vi "GetText.vi"(8 "error in":errorcluster, 11 "node in":refnum<class "Run VI Node.lvclass">) -> (0 "error out":errorcluster, 1 "additional text":string, 2 "text":string, 3 "node out":refnum<class "Run VI Node.lvclass">, 4 "glyph":string)   [LabVIEW 2014, in "Run VI Node.lvclass"]
doc: "Returns the text representation of the node used for the tree control."
uses:
  Run VI Node.lvclass
  Run VI Node.lvclass/Run VI Node.ctl
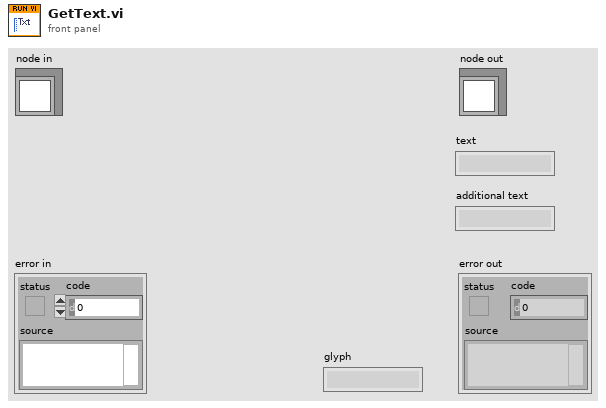
[diagram p1: front panel]
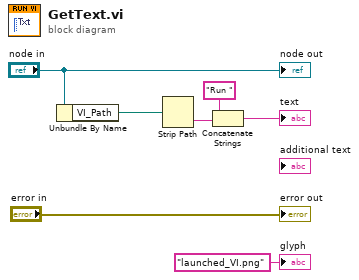
[diagram p0: block diagram]
diagram:
  n1 = Unbundle By Name("node in") -> ("VI_Path"=w5:path)
  n2 = Strip Path(path=w5) -> (name=w4:string)  [unwired: 1 out]
  n3 = Concatenate Strings("Run " ("string"), w4) -> (→"text":string)
  "error out" <- "error in"
  "node out" <- "node in"
  "glyph" <- "launched_VI.png" ("glyph")
